vi "Apply Static Header.vi"(8 "error in (no error)":errorcluster, 11 "Tx Loop Data":T1) -> (0 "error out":errorcluster, 3 "Tx Loop Data out":T1)   [LabVIEW 2016, in "UDP-Custom-Device Engine.lvlib"]
uses:
  UDP-Custom-Device Engine.lvlib
  Tx Loop Data.ctl
  <vilib>/NI Veristand/VeriStand Data/Library/Byte Buffer/Byte Buffer.lvclass
  <vilib>/NI/NIVS Inline Async API/_Data Access Engine/Data Access Engine/Types/Read.DVR.ctl
  <vilib>/NI/NIVS Inline Async API/_Data Access Engine/Access Type Classes/Read/Read.lvclass
  <vilib>/NI Veristand/VeriStand Data/Library/Typedefs/Typedefs.Data Types.ctl
  Data Conversion Config.ctl
  <vilib>/NI Veristand/VeriStand Data/Library/Byte Buffer/Byte Buffer.Mapping.ctl
  Shared/Header Details.ctl
  <vilib>/NI/NIVS Inline Async API/_Data Access Engine/Data Access Engine/Data Access Engine.lvclass
  <vilib>/NI Veristand/VeriStand Data/Library/VeriStand Data.lvlib
  Shared/UDP-Custom-Device Shared.lvlib
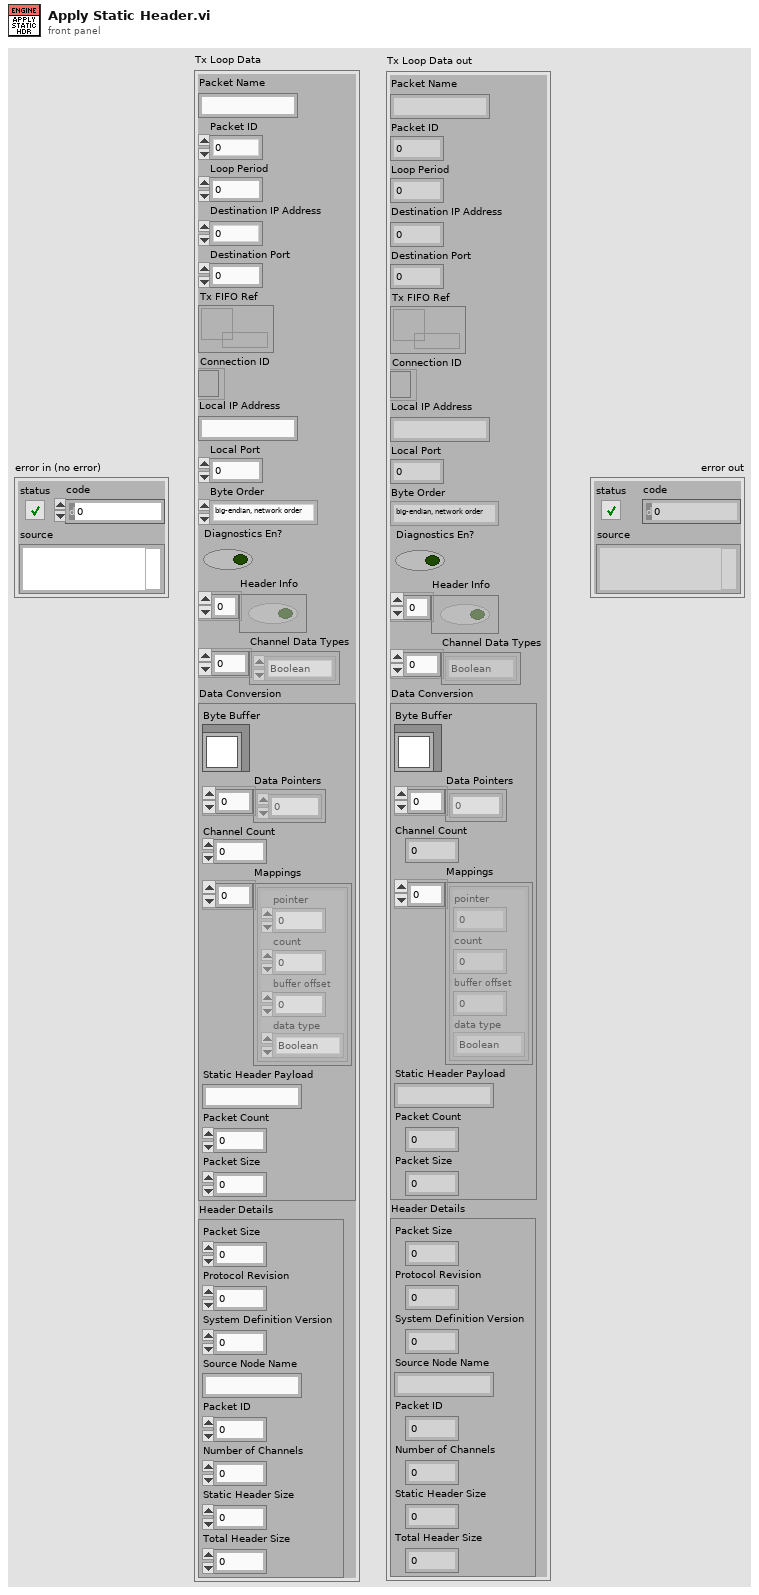
[diagram p1: front panel]
types:
  T1 = typedef "UDP-Custom-Device Engine.lvlib/Tx Loop Data.ctl" = cluster{"Packet Name":string, "Packet ID":i32, "Loop Period":u32, "Destination IP Address":u32, "Destination Port":u16, "Tx FIFO Ref":T2, "Connection ID":refnum<k16>, "Local IP Address":string, "Local Port":i32, "Byte Order":enum16{"big-endian, network order", "native, host order", "little-endian"}, "Diagnostics En?":bool, "Header Info":bool[], "Channel Data Types":T3[], "Data Conversion":T4, "Header Details":T6}
  T2 = typedef "Data Access Engine.lvlib/Data Access Engine.lvclass/Read.DVR.ctl" = refnum<data-value>
  T3 = typedef "VeriStand Data.lvlib/Typedefs.Data Types.ctl" = enum16{"Boolean", "Single", "Double", "I8", "I16", "I32", "I64", "U8", "U16", "U32", "U64"}
  T4 = typedef "UDP-Custom-Device Engine.lvlib/Data Conversion Config.ctl" = cluster{"Byte Buffer":refnum<class "Byte Buffer.lvclass">, "Data Pointers":u64[], "Channel Count":i32, "Mappings":T5[], "Static Header Payload":string, "Packet Count":dbl, "Packet Size":i32}
  T5 = typedef "VeriStand Data.lvlib/Byte Buffer.lvclass/Byte Buffer.Mapping.ctl" = cluster{"pointer":u64, "count":i32, "buffer offset":i32, "data type":T3}
  T6 = typedef "UDP-Custom-Device Shared.lvlib/Header Details.ctl" = cluster{"Packet Size":u16, "Protocol Revision":u8, "System Definition Version":u64, "Source Node Name":string, "Packet ID":u32, "Number of Channels":u32, "Static Header Size":u16, "Total Header Size":u16}
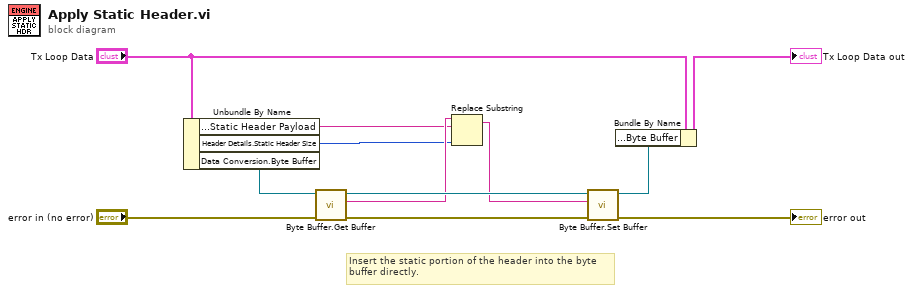
[diagram p0: block diagram]
diagram:
  # "Insert the static portion of the header into the byte\nbuffer directly."
  n1 = Unbundle By Name("Tx Loop Data") -> ("Data Conversion.Static Header Payload"=w3:string, "Header Details.Static Header Size"=w2:u16, "Data Conversion.Byte Buffer"=w12:refnum<class "Byte Buffer.lvclass">)
  n2 = call <vilib>:"Byte Buffer.Get Buffer.vi"("error in (no error)"="error in (no error)", "Byte Buffer in"=w12) -> ("error out"=w9:errorcluster, "buffer"=w4:string, "Byte Buffer out"=w10:refnum<class "Byte Buffer.lvclass">)  [unwired: 7 in]
  n3 = Replace Substring(2:w2, 4:w3, 5:w4) -> (1:w1:string)  [unwired: 1 in, 1 out]
  n4 = call <vilib>:"Byte Buffer.Set Buffer.vi"("error in (no error)"=w9, "buffer"=w1, "Byte Buffer in"=w10) -> ("error out"=→"error out":errorcluster, "Byte Buffer out"=w5:refnum<class "Byte Buffer.lvclass">)  [unwired: 7 in]
  n5 = Bundle By Name(cluster="Tx Loop Data", "Data Conversion.Byte Buffer"=w5) -> (→"Tx Loop Data out":T1)
